vi "Initialize Report Actor Core.vi"(8 "error in (no error)":errorcluster, 10 "Cluster":T1, 11 "Results in":refnum<class "Results.lvclass">) -> (0 "error out":errorcluster, 2 "stop event":refnum<user-event>, 3 "Results out":refnum<class "Results.lvclass">)   [LabVIEW 2017, in "Result Actor.lvlib" / "Results.lvclass"]
uses:
  Results.lvclass
  Results.lvclass/Results.ctl
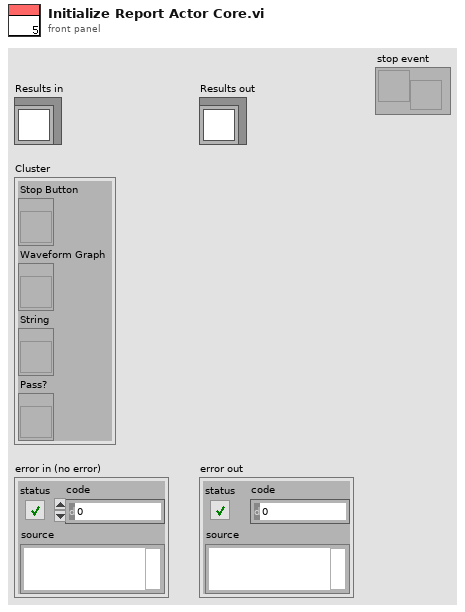
[diagram p1: front panel]
types:
  T1 = cluster{"Stop Button":refnum<vi>, "Waveform Graph":refnum<vi>, "String":refnum<vi>, "Pass?":refnum<vi>}
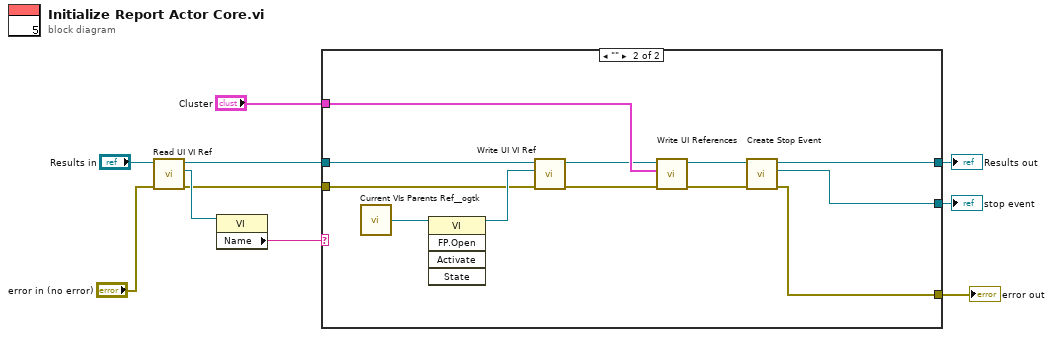
[diagram p0: block diagram]
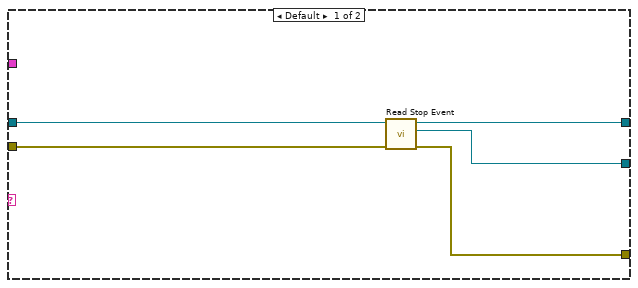
[diagram p2: hidden frame]
diagram:
  n1 = call "Read UI VI Ref.vi"("error in (no error)"="error in (no error)", "Results in"="Results in") -> ("error out"=w3:errorcluster, "UI VI Ref"=w5:refnum<vi>, "Results out"=w6:refnum<class "Results.lvclass">)  [unwired: 7 in]
  n2 = property class="VI"(reference=w5) -> ("Name"=w4:string)  [unwired: 1 in, 2 out]
  n3 = case shown="\"\"" w4 {
    tunnel: [w14 w26] -> w10
    tunnel: [w11 w25] -> w9
    tunnel: [w13 w22] -> w1
    tunnel: w6 -> [w14 w19]
    tunnel: "Cluster" -> [_ w21]
    tunnel: w3 -> [w12 w16]
    frame Default {
      n4 = call "Read Stop Event.vi"("error in (no error)"=w12, "Results in"=w14) -> ("error out"=w11:errorcluster, "stop event"=w13:refnum<user-event>)  [unwired: 7 in, 1 out]
    }
    frame "" {
      n5 = call <userlib>:"Current VIs Parents Ref__ogtk.vi"() -> ("Calling VI's Reference"=w20:refnum<vi>)  [unwired: 2 in]
      n6 = invoke class="VI" method="FP.Open"(reference=w20) -> (reference out=w17:refnum<vi>)  [unwired: 4 in, 4 out]
      n7 = call "Write UI VI Ref.vi"("error in (no error)"=w16, "UI VI Ref"=w17, "Results in"=w19) -> ("error out"=w15:errorcluster, "Results out"=w18:refnum<class "Results.lvclass">)  [unwired: 7 in]
      n8 = call "Write UI References.vi"("error in (no error)"=w15, "UI References"=w21, "Results in"=w18) -> ("error out"=w24:errorcluster, "Results out"=w23:refnum<class "Results.lvclass">)  [unwired: 7 in]
      n9 = call "Create Stop Event.vi"("error in (no error)"=w24, "Results in"=w23) -> ("error out"=w25:errorcluster, "stop event"=w22:refnum<user-event>, "Results out"=w26:refnum<class "Results.lvclass">)  [unwired: 7 in]
    }
  }
  "Results out" <- w10
  "error out" <- w9
  "stop event" <- w1
